vi "Shooter Command Handler Test.vi"(6 "Operator POVs":i16[](array[numeric]), 7 "Driver POVs":i16[](array[numeric]), 8 "Operator Axes":dbl[](array[numeric]), 9 "Operator Buttons":bool[](array[boolean]), 10 "Driver Buttons":bool[](array[boolean]), 11 "Driver Axes":dbl[](array[numeric])) -> ()   [LabVIEW 2019]
uses:
  f635170a-29a0-4b75-9924-b6fb82fe5f00.vi
  3660c45e-8d06-4759-b420-da32e730bfde.vi
  88dd05ec-de62-4f5d-9eec-dca1900521da.vi
  e0ba3985-9b44-40e8-9783-06bc49dba715.vi
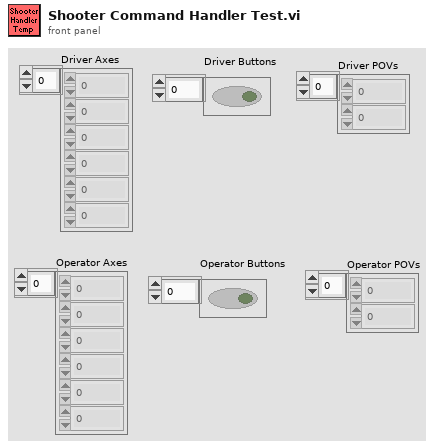
[diagram p1: front panel]
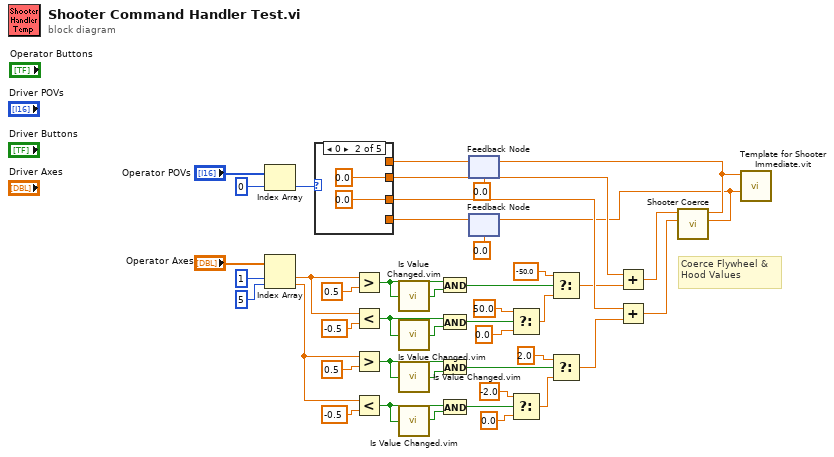
[diagram p0: block diagram]
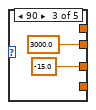
[diagram p3: hidden frame]
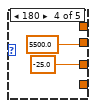
[diagram p4: hidden frame]
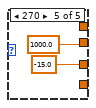
[diagram p5: hidden frame]
diagram:
  # "Coerce Flywheel & Hood Values"
  n1 = Index Array(array="Operator POVs", index=0) -> (element=w42:i16)
  n2 = Index Array(array="Operator Axes", index #1=1 ("index"), index #2=5 ("index")) -> (element #1=w36:dbl, element #2=w25:dbl)
  n3 = Greater?(x=w36, y=0.5) -> (0:w11:bool)
  n4 = Less?(x=w36, y=-0.5) -> (x < y?=w2:bool)
  n5 = Greater?(x=w25, y=0.5) -> (0:w8:bool)
  n6 = Less?(x=w25, y=-0.5) -> (x < y?=w5:bool)
  n7 = call "Is Value Changed.vim"("value"=w11) -> ("changed or first call?"=w12:bool)
  n8 = call "Is Value Changed.vim"("value"=w2) -> ("changed or first call?"=w3:bool)
  n9 = call "Is Value Changed.vim"("value"=w8) -> ("changed or first call?"=w9:bool)
  n10 = call "Is Value Changed.vim"("value"=w5) -> ("changed or first call?"=w7:bool)
  n11 = And(x=w11, y=w12) -> (x .and. y?=w10:bool)
  n12 = And(x=w2, y=w3) -> (x .and. y?=w1:bool)
  n13 = And(x=w8, y=w9) -> (x .and. y?=w6:bool)
  n14 = And(x=w5, y=w7) -> (x .and. y?=w4:bool)
  n15 = feedback #1(0.0) -> (w19:dbl)
  n16 = feedback #2(0.0) -> (w17:dbl)
  n17 = case shown="0" w42 {
    tunnel: [w45 0.0 ("Hood Setpoint") -15.0 ("Hood Setpoint") -25.0 ("Hood Setpoint") -15.0 ("Hood Setpoint")] -> w24
    tunnel: [w46 0.0 ("Flywheel Setpoint") 3000.0 ("Flywheel Setpoint") 5500.0 ("Flywheel Setpoint") 1000.0 ("Flywheel Setpoint")] -> w22
    tunnel: w19 -> [w46 _ _ _ _]
    tunnel: w17 -> [w45 _ _ _ _]
    frame -1, Default {
    }
    frame 0 {
    }
    frame 90 {
    }
    frame 180 {
    }
    frame 270 {
    }
  }
  n18 = Select(t=50.0, s=w1, f=0.0) -> (s? t:f=w32:dbl)
  n19 = Select(t=-2.0, s=w4, f=0.0) -> (s? t:f=w31:dbl)
  n20 = Select(t=-50.0, s=w10, f=w32) -> (s? t:f=w21:dbl)
  n21 = Select(t=2.0, s=w6, f=w31) -> (s? t:f=w23:dbl)
  n22 = Add(x=w22, y=w21) -> (x+y=w16:dbl)
  n23 = Add(x=w24, y=w23) -> (x+y=w15:dbl)
  n24 = call "Shooter Coerce.vi"("Hood Setpoint"=w15, "Flywheel Setpoint"=w16) -> ("Coerced Hood"=w13:dbl, "Coerced Flywheel"=w14:dbl)  [unwired: 8 in]
  n25 = feedback-in #1(w14) -> ()
  n26 = feedback-in #2(w13) -> ()
  n27 = call "Template for Shooter Immediate.vit"("Hood Setpoint"=w13, "Flywheel Setpoint"=w14) -> ()  [unwired: 9 in, 1 out]
